vi "collectTrunkGraphinfo.vi"() -> (0 "CurrentPttrunk":cluster{dbl[], dbl[]}, 1 "Centertrunk":cluster{dbl[], dbl[]}, 2 "xyboundstrunk":cluster{dbl[], dbl[]})   [LabVIEW 2024]
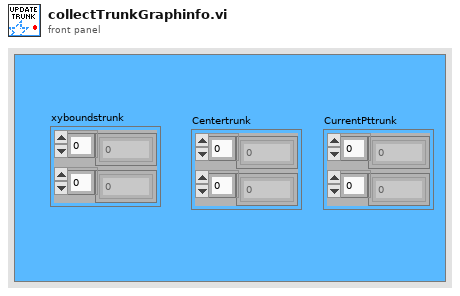
[diagram p1: front panel]
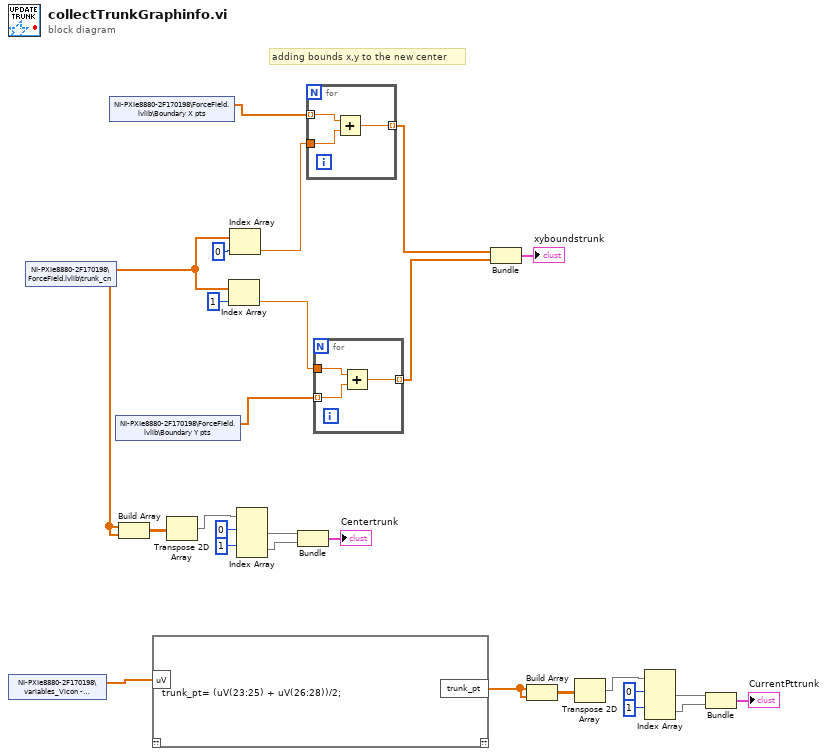
[diagram p0: block diagram]
diagram:
  # "adding bounds x,y to the new center"
  n1 = shared-variable "NI-PXIe8880-2F170198\\variables_Vicon - networkPublished.lvlib\\viconData"() -> (w9:dbl[])  [unwired: 1 in, 1 out]
  n2 = shared-variable "NI-PXIe8880-2F170198\\ForceField.lvlib\\trunk_cn"() -> (w11:dbl[])  [unwired: 1 in, 1 out]
  n3 = shared-variable "NI-PXIe8880-2F170198\\ForceField.lvlib\\Boundary X pts"() -> (w23:dbl[])  [unwired: 1 in, 1 out]
  n4 = shared-variable "NI-PXIe8880-2F170198\\ForceField.lvlib\\Boundary Y pts"() -> (w21:dbl[])  [unwired: 1 in, 1 out]
  n5 = Build Array(w11, w11) -> (w17:dbl[][])
  n6 = mathscript code="trunk_pt= (uV(23:25) + uV(26:28))/2;"("uV"=w9) -> ("trunk_pt"=w1:dbl[])  [unwired: 1 in, 1 out]
  n7 = Transpose 2D Array(2D array=w17) -> (transposed array=w15:dbl[][])
  n8 = Index Array(array=w11, index=1) -> (element=w22:dbl)
  n9 = Index Array(array=w11, index=0) -> (element=w24:dbl)
  n10 = Index Array(array=w15, index (row) #1=0 ("index (row)"), index (row) #2=1 ("index (row)")) -> (element #1=w13:dbl[], element #2=w12:dbl[])  [unwired: 2 in]
  n11 = Bundle(w13, w12) -> (→"Centertrunk":cluster{dbl[], dbl[]})  [unwired: 1 in]
  n12 = for {
    tunnel: w24 -> [w29]
    tunnel: w23 -> [w28] mode=indexing
    tunnel: [w27] -> w20 mode=indexing
    n13 = Add(x=w28, y=w29) -> (x+y=w27:dbl)
  }
  n14 = for {
    tunnel: w21 -> [w32] mode=indexing
    tunnel: w22 -> [w31]
    tunnel: [w30] -> w19 mode=indexing
    n15 = Add(x=w31, y=w32) -> (x+y=w30:dbl)
  }
  n16 = Bundle(w20, w19) -> (→"xyboundstrunk":cluster{dbl[], dbl[]})  [unwired: 1 in]
  n17 = Build Array(w1, w1) -> (w8:dbl[][])
  n18 = Transpose 2D Array(2D array=w8) -> (transposed array=w6:dbl[][])
  n19 = Index Array(array=w6, index (row) #1=0 ("index (row)"), index (row) #2=1 ("index (row)")) -> (element #1=w4:dbl[], element #2=w3:dbl[])  [unwired: 2 in]
  n20 = Bundle(w4, w3) -> (→"CurrentPttrunk":cluster{dbl[], dbl[]})  [unwired: 1 in]
